vi "조건적 자동인덱싱.vi"() -> ()   [LabVIEW 2014]
panel:
  out "웨이브폼 그래프 2":dbl[](graph)
  out "웨이브폼 그래프":dbl[](graph)
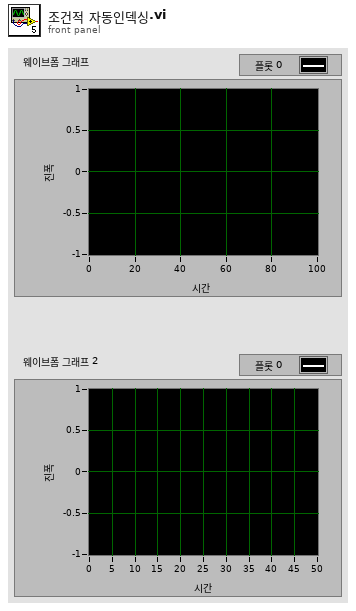
[diagram p1: front panel]
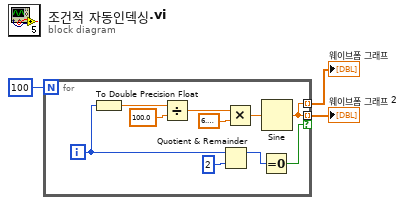
[diagram p0: block diagram]
diagram:
  n1 = for {
    N: 100 -> [_]
    tunnel: [w8] -> w2 mode=indexing
    tunnel: [w8] -> w1 mode=indexing if=w5
    i -> [w7]
    n2 = To Double Precision Float(number=w7) -> (double precision float=w13:dbl)
    n3 = Divide(x=w13, y=100.0) -> (x/y=w11:dbl)
    n4 = Quotient & Remainder(x=w7, y=2) -> (x-y*floor(x/y)=w4:i32)  [unwired: 1 out]
    n5 = Multiply(x=w11, y=6.283185307179586) -> (x*y=w9:dbl)
    n6 = Equal To 0?(x=w4) -> (x = 0?=w5:bool)
    n7 = Sine(x=w9) -> (sin(x)=w8:dbl)
  }
  "웨이브폼 그래프" <- w2
  "웨이브폼 그래프 2" <- w1
